vi "setSerializedData.vi"(0 "reference":refnum<class "SegmentedLineEdge.lvclass">, 1 "startNode":refnum<class "AbstractNode.lvclass">, 2 "endNode":refnum<class "AbstractNode.lvclass">, 3 "xmlOut":string, 5 "error in (no error)":errorcluster) -> (14 "reference out":refnum<class "SegmentedLineEdge.lvclass">, 19 "error out":errorcluster)   [LabVIEW 2012, in "SegmentedLineEdge.lvclass"]
doc: "setSerializedData"
uses:
  <resource>/Framework/Providers/Open_GDS/UML/SegmentedLineEdge_class/SegmentedLineEdge.lvclass
  <resource>/Framework/Providers/Open_GDS/UML/AbstractNode_class/AbstractNode.lvclass
  <resource>/Framework/Providers/Open_GDS/UML/AbstractNode_class/ObjectReference.ctl
  <resource>/Framework/Providers/Open_GDS/UML/LineStyle_class/ObjectReference.ctl
  <resource>/Framework/Providers/Open_GDS/UML/ArrowHead_class/ObjectReference.ctl
  <resource>/Framework/Providers/Open_GDS/UML/General/Point/Point Point2D.ctl
  <resource>/Framework/Providers/Open_GDS/UML/LineStyle_class/LineStyleType.ctl
  <resource>/Framework/Providers/Open_GDS/UML/ArrowHead_class/ArrowHeadType.ctl
  <resource>/Framework/Providers/Open_GDS/UML/LineStyle_class/LineStyle.lvclass
  <resource>/Framework/Providers/Open_GDS/UML/ArrowHead_class/ArrowHead.lvclass
  <resource>/Framework/Providers/Open_GDS/UML/AbstractEdge_class/AbstractEdge.lvclass
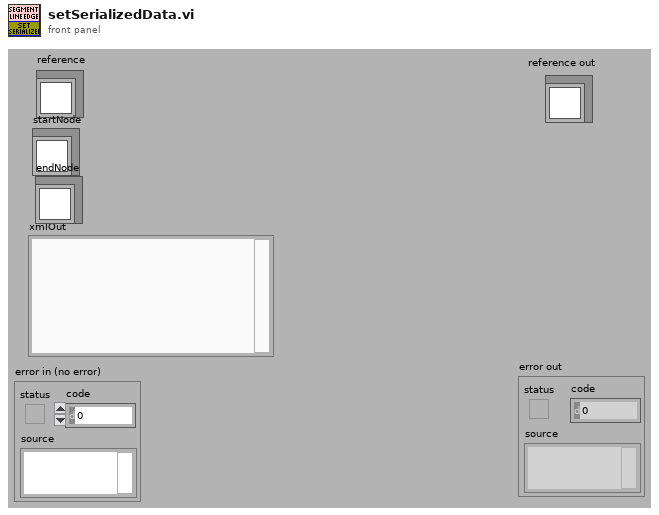
[diagram p1: front panel]
types:
  T1 = typedef "AbstractNode.lvclass/ObjectReference.ctl" = refnum<k1>
  T2 = typedef "LineStyle.lvclass/ObjectReference.ctl" = refnum<k1>
  T3 = typedef "ArrowHead.lvclass/ObjectReference.ctl" = refnum<k1>
  T4 = typedef "Point Point2D.ctl" = cluster{"x":dbl, "y":dbl}
  T5 = cluster{"Base class":cluster{"Base class":cluster{"start":T1, "end":T1}}, "lineStyle":T2, "startArrowHead":T3, "endArrowHead":T3, "startLabel":string, "midLabel":string, "endLabel":string, "MidLabelOffset":T4}
  T6 = cluster{"Base class":cluster{"Base class":cluster{"start":T1, "end":T1}}, "lineStyle":T2, "startArrowHead":T3, "endArrowHead":T3, "startLabel":string, "midLabel":string, "endLabel":string, "MidLabelOffset":T4, "SplitWire":bool}
  T7 = typedef "LineStyle.lvclass/LineStyleType.ctl" = enum16{"SOLID", "DOTTED"}
  T8 = typedef "ArrowHead.lvclass/ArrowHeadType.ctl" = enum16{"NONE", "TRIANGLE", "BLACK_TRIANGLE", "V", "HALF_V", "DIAMOND", "BLACK_DIAMOND"}
  T9 = cluster{"Base class":cluster{"Base class":cluster{"Base class":cluster{"start":T1, "end":T1}}, "lineStyle":T2, "startArrowHead":T3, "endArrowHead":T3, "startLabel":string, "midLabel":string, "endLabel":string, "MidLabelOffset":T4}, string, string, string}
  T10 = cluster{"Base class":cluster{"Base class":cluster{"Base class":cluster{"start":T1, "end":T1}}, "lineStyle":T2, "startArrowHead":T3, "endArrowHead":T3, "startLabel":string, "midLabel":string, "endLabel":string, "MidLabelOffset":T4, "SplitWire":bool}, string, string, string}
  T11 = typedef "AbstractEdge.lvclass/ObjectAttributes.ctl" = cluster{"start":refnum<class "AbstractNode.lvclass">, "end":refnum<class "AbstractNode.lvclass">}
  T12 = typedef "SegmentedLineEdge.lvclass/ObjectAttributes.ctl" = cluster{"lineStyle":refnum<class "LineStyle.lvclass">, "startArrowHead":refnum<class "ArrowHead.lvclass">, "endArrowHead":refnum<class "ArrowHead.lvclass">, "startLabel":string, "midLabel":string, "endLabel":string, "MidLabelOffset":T4, "SplitWire":bool}
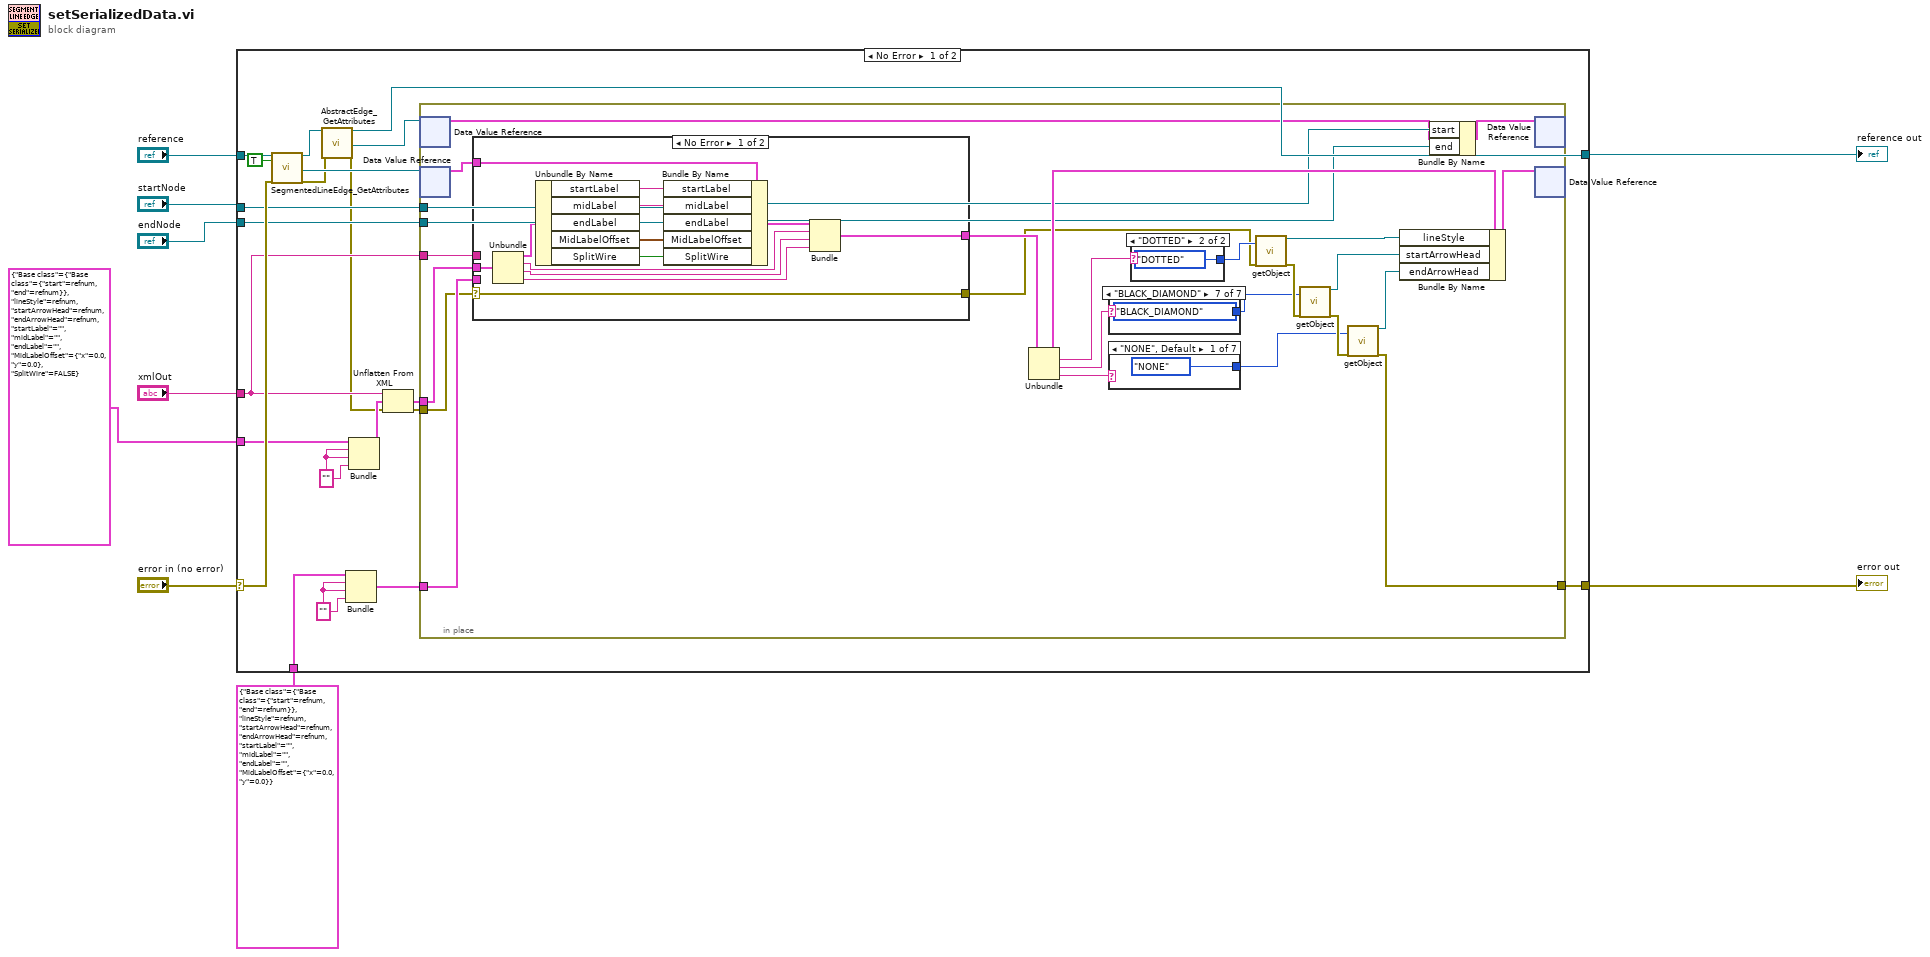
[diagram p0: block diagram]
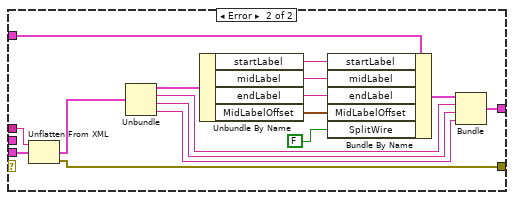
[diagram p2: hidden frame]
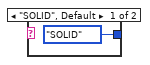
[diagram p3: hidden frame]
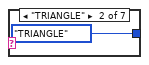
[diagram p4: hidden frame]
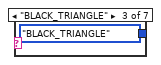
[diagram p5: hidden frame]
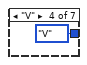
[diagram p6: hidden frame]
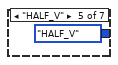
[diagram p7: hidden frame]
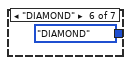
[diagram p8: hidden frame]
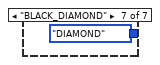
[diagram p9: hidden frame]
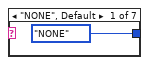
[diagram p10: hidden frame]
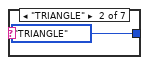
[diagram p11: hidden frame]
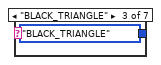
[diagram p12: hidden frame]
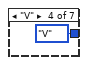
[diagram p13: hidden frame]
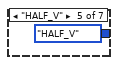
[diagram p14: hidden frame]
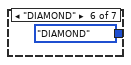
[diagram p15: hidden frame]
diagram:
  n1 = case shown="No Error" "error in (no error)" {
    selector: "error in (no error)" -> [w29 w102]
    tunnel: "reference" -> [w30 w103]
    tunnel: [w11 w103] -> w7
    tunnel: [w28 w102] -> w6
    tunnel: "xmlOut" -> [w19 _]
    tunnel: "startNode" -> [w27 _]
    tunnel: "endNode" -> [w26 _]
    tunnel: T5 {"Base class"={"Base class"={"start"=refnum, "end"=refnum}}, "lineStyle"=refnum, "startArrowHead"=refnum, "endArrowHead"=refnum, "startLabel"="", "midLabel"="", "endLabel"="", "MidLabelOffset"={"x"=0.0, "y"=0.0}} ("Base class") -> [w23 _]
    tunnel: T6 {"Base class"={"Base class"={"start"=refnum, "end"=refnum}}, "lineStyle"=refnum, "startArrowHead"=refnum, "endArrowHead"=refnum, "startLabel"="", "midLabel"="", "endLabel"="", "MidLabelOffset"={"x"=0.0, "y"=0.0}, "SplitWire"=FALSE} ("Base class") -> [w22 _]
    frame No Error {
      w24 = ""
      w25 = ""
      n2 = call <resource>:"SegmentedLineEdge_GetAttributes.vi"("reference in"=w30, "OnlyGetDvrReference(False)"=TRUE, "error in (no error)"=w29) -> ("reference out"=w12:refnum<class "SegmentedLineEdge.lvclass">, "DataRef"=w15:refnum<data-value>, "error out"=w14:errorcluster)  [unwired: 13 in, 1 out]
      n3 = call <resource>:"AbstractEdge_GetAttributes.vi"("reference in"=w12, "error in (no error)"=w14) -> ("reference out"=w11:refnum<class "SegmentedLineEdge.lvclass">, "DataRef"=w10:refnum<data-value>, "error out"=w13:errorcluster)  [unwired: 14 in, 1 out]
      n4 = Bundle("Base class"=w23, w24, w24, w24) -> (w18:T9)  [unwired: 1 out]
      n5 = Bundle("Base class"=w22, w25, w25, w25) -> (w17:T10)  [unwired: 1 out]
      n6 = Unflatten From XML(xml string=w19, type=w17, error in (no error)=w13) -> (value=w20:T10, error out=w16:errorcluster)
      n7 = in-place {
        in-place-border: [w49] -> w28
        in-place-border: w27 -> [w34]
        in-place-border: w26 -> [w33]
        in-place-border: w20 -> [w42]
        in-place-border: w19 -> [w41]
        in-place-border: w18 -> [w40]
        in-place-border: w16 -> [w37]
        n8 = in-place-dvr #1(w10) -> (w32:T11)  [unwired: 1 out]
        n9 = in-place-dvr #2(w15) -> (w36:T12)  [unwired: 1 out]
        n10 = case shown="No Error" w37 {
          selector: w37 -> [w69 _]
          tunnel: [w64 w81] -> w39
          tunnel: w42 -> [w68 _]
          tunnel: [w69 w83] -> w38
          tunnel: w41 -> [_ w85]
          tunnel: w40 -> [_ w84]
          tunnel: w36 -> [w57 w74]
          frame No Error {
            n11 = Unbundle(w68) -> ("Base class"=w58:T6, w65:string, w66:string, w67:string)
            n12 = Unbundle By Name(w58) -> ("startLabel"=w63:string, "midLabel"=w62:string, "endLabel"=w61:string, "MidLabelOffset"=w60:T4, "SplitWire"=w59:bool)
            n13 = Bundle By Name(cluster=w57, "startLabel"=w63, "midLabel"=w62, "endLabel"=w61, "MidLabelOffset"=w60, "SplitWire"=w59) -> (w56:T12)
            n14 = Bundle("Data"=w56, w65, w66, w67) -> (w64:cluster{"Data":T12, string, string, string})  [unwired: 1 out]
          }
          frame Error {
            n15 = Unflatten From XML(xml string=w85, type=w84) -> (value=w82:T9, error out=w83:errorcluster)  [unwired: 1 in]
            n16 = Unbundle(w82) -> ("Base class"=w76:T5, w78:string, w79:string, w80:string)
            n17 = Unbundle By Name(w76) -> ("startLabel"=w72:string, "midLabel"=w71:string, "endLabel"=w70:string, "MidLabelOffset"=w77:T4)
            n18 = Bundle By Name(cluster=w74, "startLabel"=w72, "midLabel"=w71, "endLabel"=w70, "MidLabelOffset"=w77, "SplitWire"=FALSE) -> (w73:T12)
            n19 = Bundle("Data"=w73, w78, w79, w80) -> (w81:cluster{"Data":T12, string, string, string})  [unwired: 1 in]
          }
        }
        n20 = Unbundle(w39) -> ("Data"=w50:T12, w44:string, w47:string, w46:string)
        n21 = case shown="\"BLACK_DIAMOND\"" w47 {
          tunnel: [ArrowHeadType."NONE" ("arrowHead") ArrowHeadType."TRIANGLE" ("arrowHead") ArrowHeadType."BLACK_TRIANGLE" ("arrowHead") ArrowHeadType."V" ("arrowHead") ArrowHeadType."HALF_V" ("arrowHead") ArrowHeadType."DIAMOND" ("arrowHead") ArrowHeadType."BLACK_DIAMOND" ("arrowHead")] -> w48
          frame "NONE", Default {
          }
          frame "TRIANGLE" {
          }
          frame "BLACK_TRIANGLE" {
          }
          frame "V" {
          }
          frame "HALF_V" {
          }
          frame "DIAMOND" {
          }
          frame "BLACK_DIAMOND" {
          }
        }
        n22 = case shown="\"NONE\", Default" w46 {
          tunnel: [ArrowHeadType."NONE" ("arrowHead") ArrowHeadType."TRIANGLE" ("arrowHead") ArrowHeadType."BLACK_TRIANGLE" ("arrowHead") ArrowHeadType."V" ("arrowHead") ArrowHeadType."HALF_V" ("arrowHead") ArrowHeadType."DIAMOND" ("arrowHead") ArrowHeadType."DIAMOND" ("arrowHead")] -> w45
          frame "NONE", Default {
          }
          frame "TRIANGLE" {
          }
          frame "BLACK_TRIANGLE" {
          }
          frame "V" {
          }
          frame "HALF_V" {
          }
          frame "DIAMOND" {
          }
          frame "BLACK_DIAMOND" {
          }
        }
        n23 = case shown="\"DOTTED\"" w44 {
          tunnel: [LineStyleType."SOLID" ("lineStyle") LineStyleType."DOTTED" ("lineStyle")] -> w43
          frame "SOLID", Default {
          }
          frame "DOTTED" {
          }
        }
        n24 = call <resource>:"getObject.vi"("lineStyle"=w43, "error in (no error)"=w38) -> ("reference out"=w55:refnum<class "LineStyle.lvclass">, "error out"=w54:errorcluster)  [unwired: 16 out]
        n25 = call <resource>:"getObject.vi"("arrowHead"=w48, "error in (no error)"=w54) -> ("reference out"=w51:refnum<class "ArrowHead.lvclass">, "error out"=w53:errorcluster)  [unwired: 16 out]
        n26 = call <resource>:"getObject.vi"("arrowHead"=w45, "error in (no error)"=w53) -> ("reference out"=w52:refnum<class "ArrowHead.lvclass">, "error out"=w49:errorcluster)  [unwired: 16 out]
        n27 = Bundle By Name(cluster=w50, "lineStyle"=w55, "startArrowHead"=w51, "endArrowHead"=w52) -> (w35:T12)
        n28 = Bundle By Name(cluster=w32, "start"=w34, "end"=w33) -> (w31:T11)
        n29 = in-place-dvr #1(w31) -> ()  [unwired: 2 out]
        n30 = in-place-dvr #2(w35) -> ()  [unwired: 2 out]
      }
    }
    frame Error {
    }
  }
  "reference out" <- w7
  "error out" <- w6
